vi "Status Pump Status.vi"(5 "Retry Attempts (0)":i32 min=0, 7 "Fast Comms (F)":bool, 8 "error in (no error)":errorcluster, 11 "VISA resource name":refnum<visa-resource-name>) -> (0 "error out":errorcluster, 2 "Status Cluster":T1, 3 "VISA resource name out":refnum<visa-resource-name>)   [LabVIEW 2020, in "ChromTech MX-Class Drivers.lvlib"]
doc: "Returns the current pump information."
uses:
  <instrlib>/RxnRover/ChromtechNextGenDriver/ChromTech MX-Class Drivers.lvlib
panel:
  out "Response":string
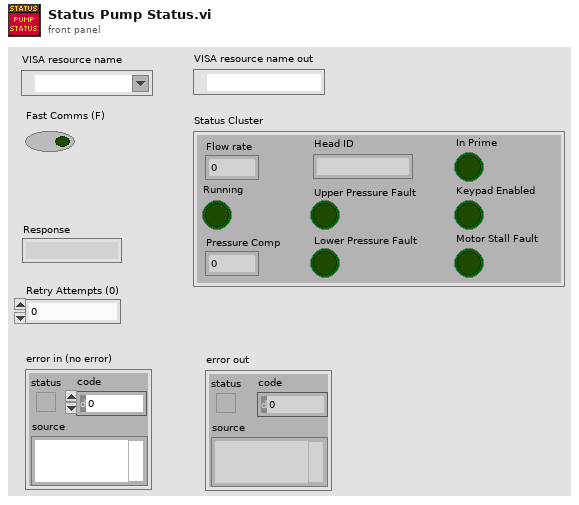
[diagram p1: front panel]
types:
  T1 = cluster{"Flow rate":dbl, "Running":bool, "Pressure Comp":i32, "Head ID":string, "Upper Pressure Fault":bool, "Lower Pressure Fault":bool, "In Prime":bool, "Keypad Enabled":bool, "Motor Stall Fault":bool}
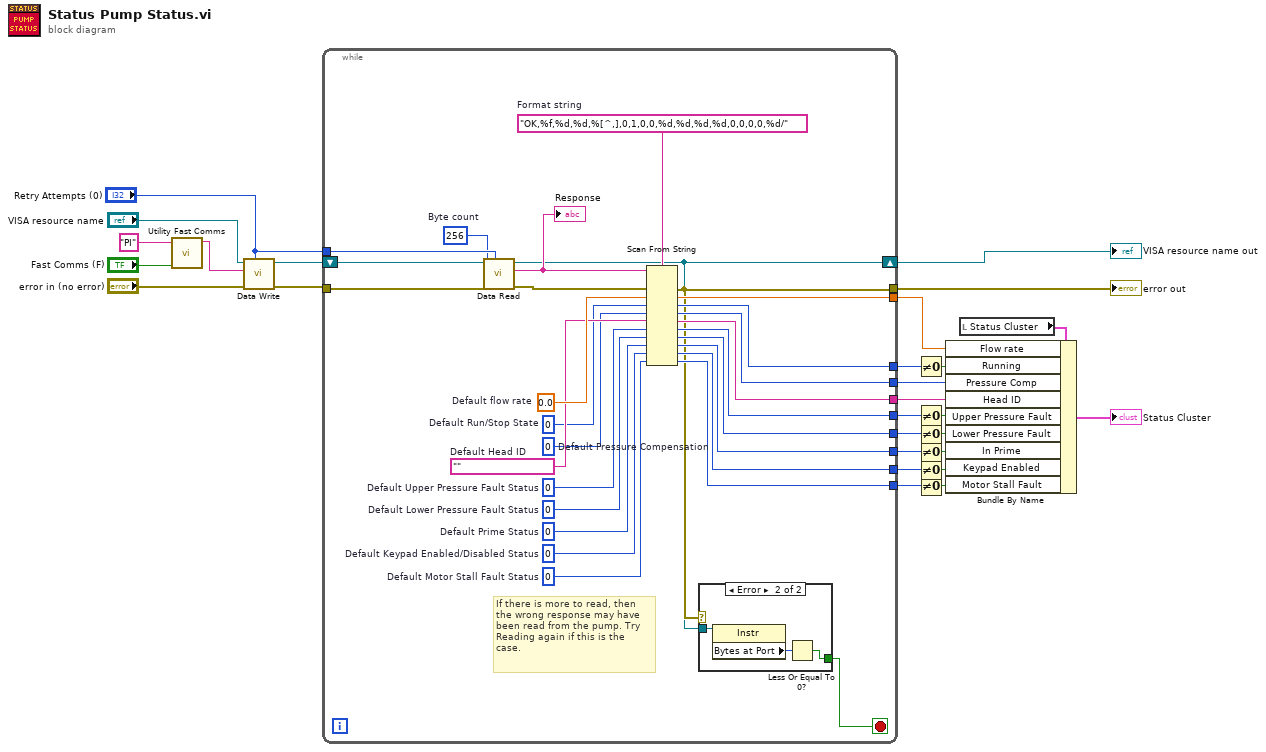
[diagram p0: block diagram]
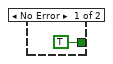
[diagram p2: hidden frame]
diagram:
  n1 = call <instrlib>:"Utility Fast Comms.vi"("Fast Comms"="Fast Comms (F)", "Command"="PI" ("command")) -> ("Fast Command"=w23:string)  [unwired: 9 in]
  n2 = call <instrlib>:"Data Write.vi"("Retry Attempts (0)"="Retry Attempts (0)", "error in (no error)"="error in (no error)", "Command"=w23, "VISA Refnum in"="VISA resource name") -> ("error out"=w4:errorcluster, "VISA Refnum out"=w3:refnum<visa-resource-name>)  [unwired: 6 in]
  n3 = while {
    tunnel: [w49] -> w20
    tunnel: [w48] -> w13
    tunnel: [w47] -> w12
    tunnel: [w46] -> w11
    tunnel: [w45] -> w10
    tunnel: [w44] -> w9
    tunnel: [w43] -> w8
    tunnel: [w42] -> w7
    tunnel: [w41] -> w6
    tunnel: "Retry Attempts (0)" -> [w34]
    shift-right: [w29] -> w1
    shift-left: w3 -> [w31]
    tunnel: w4 -> [w33]
    tunnel: [w30] -> w2
    stop <- w28 stop-if-true
    w32 = u32 256  # Byte count
    w37 = 0  # Default Motor Stall Fault Status
    w38 = 0  # Default Keypad Enabled/Disabled Status
    w39 = 0  # Default Prime Status
    w40 = 0  # Default Lower Pressure Fault Status
    w50 = 0  # Default Pressure Compensation
    w51 = 0  # Default Run/Stop State
    w52 = 0  # Default Upper Pressure Fault Status
    w53 = ""  # Default Head ID
    w54 = 0.0  # Default flow rate
    w55 = "OK,%f,%d,%d,%[^,],0,1,0,0,%d,%d,%d,%d,0,0,0,0,%d/"  # Format string
    # "If there is more to read, then\nthe wrong response may have\nbeen read from the pump. Try\nReading again if this is the\ncase."
    n4 = call <instrlib>:"Data Read.vi"("Retry Attempts (0)"=w34, "error in (no error)"=w33, "Bytes to read"=w32, "VISA Refnum in"=w31) -> ("error out"=w36:errorcluster, "read buffer"=w35:string, "VISA Refnum out"=w29:refnum<visa-resource-name>)  [unwired: 5 in]
    "Response" <- w35
    n5 = Scan From String(format string=w55, input string=w35, error in=w36, default 1=w54, default 2=w51, default 3=w50, default 4=w53, default 5=w52, default 6=w40, default 7=w39, default 8=w38, default 9=w37) -> (error out=w30:errorcluster, output 1=w49:dbl, output 2=w48:i32, output 3=w47:i32, output 4=w46:string, output 5=w45:i32, output 6=w44:i32, output 7=w43:i32, output 8=w42:i32, output 9=w41:i32)  [unwired: 1 in, 2 out]
    n6 = case shown="Error" w30 {
      tunnel: w29 -> [_ w59]
      tunnel: [TRUE w57] -> w28
      frame No Error {
      }
      frame Error {
        n7 = property class="Instr"(reference=w59) -> ("Bytes at Port"=w58:u32)  [unwired: 1 in, 2 out]
        n8 = Less Or Equal To 0?(x=w58) -> (x <= 0?=w57:bool)
      }
    }
  }
  "VISA resource name out" <- w1
  "error out" <- w2
  n9 = Not Equal To 0?(x=w13) -> (x != 0?=w19:bool)
  n10 = Not Equal To 0?(x=w10) -> (x != 0?=w18:bool)
  n11 = Not Equal To 0?(x=w9) -> (x != 0?=w17:bool)
  n12 = Not Equal To 0?(x=w8) -> (x != 0?=w16:bool)
  n13 = Not Equal To 0?(x=w7) -> (x != 0?=w15:bool)
  n14 = Not Equal To 0?(x=w6) -> (x != 0?=w14:bool)
  n15 = local read "Status Cluster"() -> (w22:T1)
  n16 = Bundle By Name(cluster=w22, "Flow rate"=w20, "Running"=w19, "Pressure Comp"=w12, "Head ID"=w11, "Upper Pressure Fault"=w18, "Lower Pressure Fault"=w17, "In Prime"=w16, "Keypad Enabled"=w15, "Motor Stall Fault"=w14) -> (→"Status Cluster":T1)
